vi "CalculPosition.vi"   [LabVIEW 2019]
uses:
  <vilib>/Rock Robotics/WPI/ThirdParty/Sensors/navX/_TypeDefs/FRIC_navX_DeviceNumbersTypeDef.ctl
  <vilib>/Rock Robotics/WPI/ThirdParty/Phoenix-LabVIEW/Motor Controller/Get/CTRE_Phoenix_MotorController_GetQuadratureData.vi
types:
  T1 = typedef "FRIC_navX_DeviceNumbersTypeDef.ctl" = enum16{"Dev0", "Dev1", "Dev2", "Dev3"}
  T2 = cluster{"Yaw":dbl, "Roll":dbl, "Pitch":dbl, "Heading":dbl, "Fused Heading":dbl}
  T3 = typedef "WPI_MotorControlDeviceRef.ctl" = cluster{"DeviceStatus":errorcluster, "Type":T4, "PWM":cluster{"PWM Channel":T5, "DeadBand":T6}, "CAN":cluster{"Device Number":u8, "SetOutput VI Ref":variant, "GetOutput VI Ref":variant, "Enable VI Ref":variant, "Disable VI Ref":variant, "Data":variant}, "Invert":bool, "DIO PWM":cluster{"PWM \"Enable\" Channel":T5, "DIOChannel":T7, "PWM Rate":dbl}}
  T4 = typedef "WPI_MotorControlType.ctl" = enum16{"PWM", "CAN", "DIO PWM"}
  T5 = typedef "FPGA_DIOPWMChannel.ctl" = enum8{"PWM 0", "PWM 1", "PWM 2", "PWM 3", "PWM 4", "PWM 5", "PWM 6", "PWM 7", "PWM 8", "PWM 9", "PWM MXP 0", "PWM MXP 1", "PWM MXP 2", "PWM MXP 3", "PWM MXP 4", "PWM MXP 5", "PWM MXP 6", "PWM MXP 7", "PWM MXP 8", "PWM MXP 9", "Invalid"}
  T6 = typedef "WPI_PWMDeadband.ctl" = cluster{"Name":string, "maxPositivePwm":i32, "minPositivePwm":i32, "centerPwm":i32, "maxNegativePwm":i32, "minNegativePwm":i32, "angularRange":u16}
  T7 = typedef "FPGA_DIOChannel.ctl" = enum8{"DIO 0", "DIO 1", "DIO 2", "DIO 3", "DIO 4", "DIO 5", "DIO 6", "DIO 7", "DIO 8", "DIO 9", "DIO MXP 0", "DIO MXP 1", "DIO MXP 2", "DIO MXP 3", "DIO MXP 4", "DIO MXP 5", "DIO MXP 6", "DIO MXP 7", "DIO MXP 8", "DIO MXP 9", "DIO MXP 10", "DIO MXP 11", "DIO MXP 12", "DIO MXP 13", "DIO MXP 14", "DIO MXP 15", "SPI Port CS1", "SPI Port CS2", "SPI Port CS3", "SPI Port MISO", "SPI Port MOSI", "Invalid"}
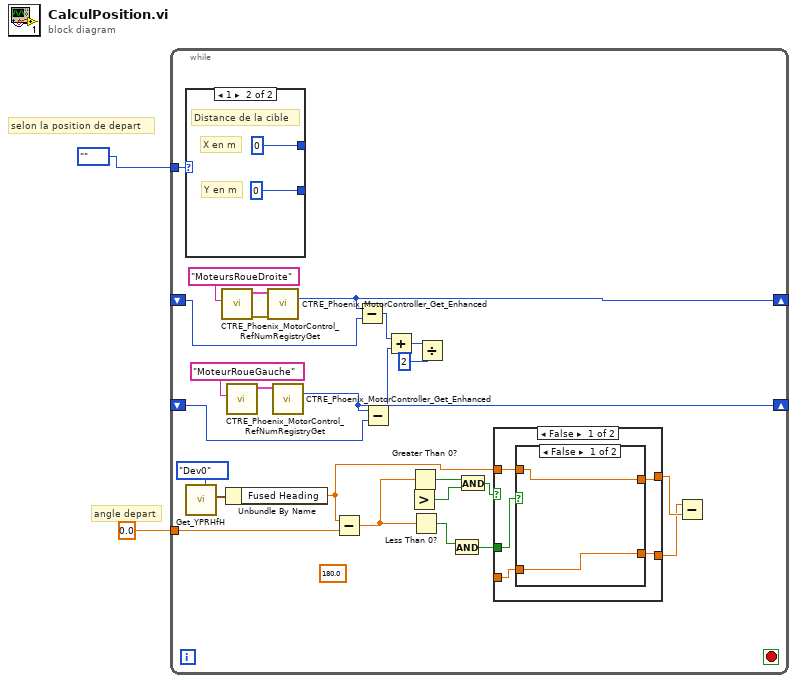
[diagram p0: block diagram]
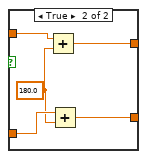
[diagram p2: hidden frame]
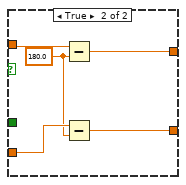
[diagram p3: hidden frame]
diagram:
  # "angle depart"
  # "selon la position de depart"
  n1 = while {
    tunnel: enum16{""}."" -> [w29]
    shift-right: [w20] -> _
    shift-left: _ -> [w18]
    shift-right: [w21] -> _
    shift-left: _ -> [w19]
    tunnel: 0.0 -> [w4]
    stop <- _ stop-if-true
    (unwired) 180.0 ("x")
    n2 = case shown="\"1\"" w29 {
      tunnel: [_ 0] -> _
      tunnel: [_ 0] -> _
      frame "", Default {
      }
      frame 1 {
        # "Distance de la cible"
        # "Y en m"
        # "X en m"
      }
    }
    n3 = call <vilib>:"Get_YPRHfH.vi"("Device Number"=FRIC_navX_DeviceNumbersTypeDef."Dev0") -> ("YRPHfH"=w27:T2)  [unwired: 10 in]
    n4 = call <vilib>:"CTRE_Phoenix_MotorControl_RefNumRegistryGet.vi"("refnum name"="MoteursRoueDroite") -> ("error out"=w26:errorcluster, "PhoenixMotorControlDevRef"=w25:T3)  [unwired: 9 in]
    n5 = Unbundle By Name(w27) -> ("Fused Heading"=w5:dbl)
    n6 = call <vilib>:"CTRE_Phoenix_MotorControl_RefNumRegistryGet.vi"("refnum name"="MoteurRoueGauche") -> ("PhoenixMotorControlDevRef"=w23:T3)  [unwired: 9 in, 1 out]
    n7 = call-poly <vilib>:"CTRE_Phoenix_MotorController_Get_Enhanced.vi"("PhoenixMotorControlDevRef"=w25, "error in"=w26) -> ("Quadrature Position"=w21:i32)  [unwired: 10 in, 3 out]
    n8 = call-poly <vilib>:"CTRE_Phoenix_MotorController_Get_Enhanced.vi"("PhoenixMotorControlDevRef"=w23) -> ("Quadrature Position"=w20:i32)  [unwired: 11 in, 3 out]
    n9 = Subtract(x=w5, y=w4) -> (x-y=w3:dbl)
    n10 = Subtract(x=w21, y=w19) -> (x-y=w17:i32)
    n11 = Subtract(x=w20, y=w18) -> (x-y=w16:i32)
    n12 = Add(x=w17, y=w16) -> (x+y=w15:i32)
    n13 = Greater?() -> (0:w11:bool)  [unwired: 2 in]
    n14 = Greater Than 0?(x=w3) -> (x > 0?=w12:bool)
    n15 = Less Than 0?(x=w3) -> (x < 0?=w13:bool)
    n16 = Divide(x=w15, y=2) -> ()  [unwired: 1 out]
    n17 = And(x=w13) -> (x .and. y?=w9:bool)  [unwired: 1 in]
    n18 = And(x=w12, y=w11) -> (x .and. y?=w10:bool)
    n19 = case shown="False" w10 {
      tunnel: w9 -> [w34 _]
      tunnel: w5 -> [w32 w45]
      tunnel: [w33 w46] -> w6
      tunnel: [w30 w43] -> w7
      tunnel: [w31 w42] -> w8
      frame False {
        n20 = case shown="False" w34 {
          tunnel: w33 -> [w36 w41]
          tunnel: w32 -> [w35 w40]
          tunnel: [w35 w38] -> w31
          tunnel: [w36 w37] -> w30
          frame False {
          }
          frame True {
            w39 = 180.0 ("y")
            n21 = Add(x=w40, y=w39) -> (x+y=w38:dbl)
            n22 = Add(x=w41, y=w39) -> (x+y=w37:dbl)
          }
        }
      }
      frame True {
        w44 = 180.0 ("y")
        n23 = Subtract(x=w45, y=w44) -> (x-y=w42:dbl)
        n24 = Subtract(x=w46, y=w44) -> (x-y=w43:dbl)
      }
    }
    n25 = Subtract(x=w7, y=w8) -> ()  [unwired: 1 out]
  }
